vi "matrix_transformation.vi"(2 "Transformation Centre":cluster{dbl, dbl, dbl}, 3 "Transformation Matrix":T1, 4 "Input Vector":cluster{dbl, dbl, dbl}) -> (0 "Output Vector":cluster{dbl, dbl, dbl})   [LabVIEW 2010]
uses:
  <vilib>/Analysis/Matrix/Datatypes/RealMatrix.ctl
  <vilib>/Analysis/Matrix/Numeric/Conversions/Array To Matrix - RA.vi
  <vilib>/Analysis/baseanly.llb/Real A x B.vi
  <vilib>/Analysis/Matrix/Numeric/Conversions/Matrix To Array - RM.vi
  <vilib>/Analysis/Matrix/NI_Matrix.lvlib
  <vilib>/Analysis/NI_AALBase.lvlib
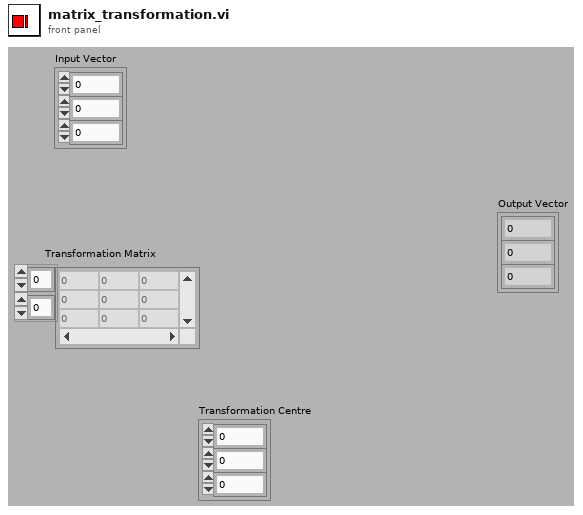
[diagram p1: front panel]
types:
  T1 = typedef "NI_Matrix.lvlib/RealMatrix.ctl" = dbl[][]
  T2 = cluster{"Real Matrix Element":dbl, "Real Matrix Element":dbl, "Real Matrix Element":dbl}
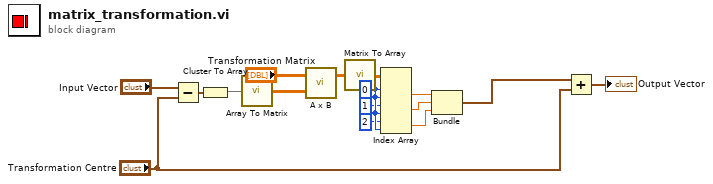
[diagram p0: block diagram]
diagram:
  w4 = 0 ("index (row)")
  n1 = Subtract(x="Input Vector", y="Transformation Centre") -> (x-y=w13:cluster{dbl, dbl, dbl})
  n2 = Cluster To Array(cluster=w13) -> (array=w12:dbl[])
  n3 = call-poly <vilib>:"Array To Matrix.vi"("Real 1D Array"=w12) -> ("Real Matrix (Column Vector)"=w11:T1)
  n4 = call-poly <vilib>:"A x B.vi"("B"=w11, "A"="Transformation Matrix") -> ("A x B"=w9:T1)  [unwired: 1 out]
  n5 = call-poly <vilib>:"Matrix To Array.vi"("Real Matrix"=w9) -> ("Real 2D Array"=w8:dbl[][])
  n6 = Index Array(array=w8, index (row) #1=w4, index (col) #1=w4, index (row) #2=1 ("disabled index (row)"), index (col) #2=w4, index (row) #3=2 ("disabled index (row)"), index (col) #3=w4) -> (element #1=w7:dbl, element #2=w6:dbl, element #3=w5:dbl)
  n7 = Bundle("Real Matrix Element"=w7, "Real Matrix Element"=w6, "Real Matrix Element"=w5) -> (w1:T2)  [unwired: 1 out]
  n8 = Add(x=w1, y="Transformation Centre") -> (x+y=→"Output Vector":cluster{dbl, dbl, dbl})
